vi "Test Assert Not Equal Value.vi"(8 "error in (no error)":errorcluster) -> (0 "error out":errorcluster)   [LabVIEW 2009]
uses:
  classes/Assert/Assert.lvclass
  classes/Test/Test.lvclass
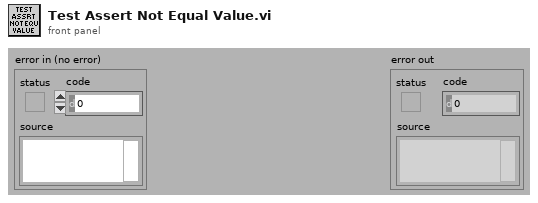
[diagram p1: front panel]
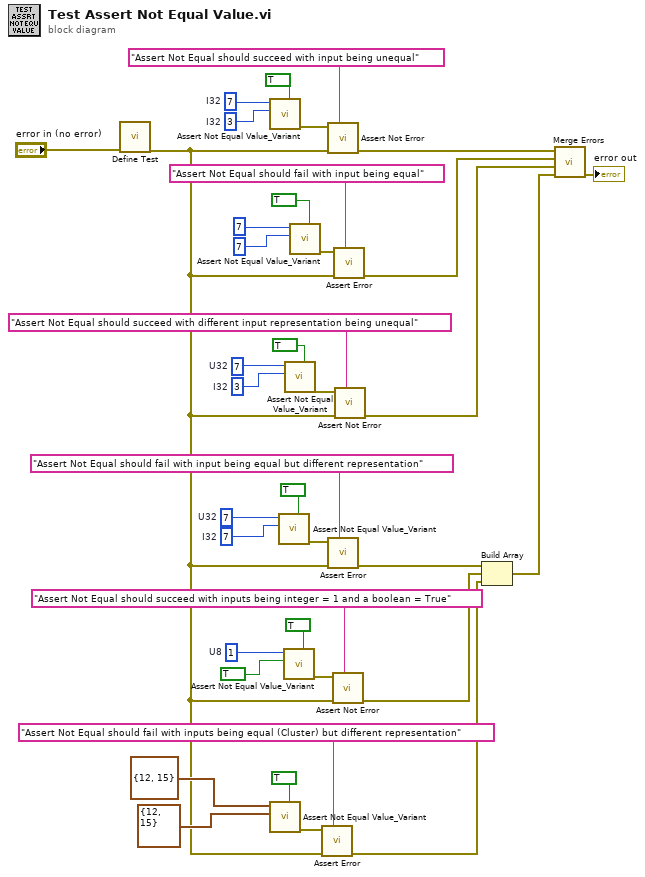
[diagram p0: block diagram]
diagram:
  w12 = u8 1  # U8
  w18 = 7  # I32
  w19 = u32 7  # U32
  w20 = 3  # I32
  w21 = u32 7  # U32
  w28 = 3  # I32
  w29 = 7  # I32
  n1 = call "Define Test.vi"("error in (no error)"="error in (no error)") -> ("error out"=w2:errorcluster)  [unwired: 10 in]
  n2 = call "Assert Not Equal Value_Variant.vi"("Assert Only? (F)"=TRUE, "Y"=w28, "X"=w29) -> ("error out"=w31:errorcluster)  [unwired: 8 in]
  n3 = call "Assert Not Equal Value_Variant.vi"("Assert Only? (F)"=TRUE, "Y"=cluster{"Width":u32, "I32":i32} {"Width"=12, "I32"=15} ("Bounds"), "X"=cluster{"Width":u32, "U32":u32} {"Width"=12, "U32"=15} ("Bounds")) -> ("error out"=w6:errorcluster)  [unwired: 8 in]
  n4 = call "Assert Not Equal Value_Variant.vi"("Assert Only? (F)"=TRUE, "Y"=w18, "X"=w19) -> ("error out"=w15:errorcluster)  [unwired: 8 in]
  n5 = call "Assert Not Equal Value_Variant.vi"("Assert Only? (F)"=TRUE, "Y"=TRUE, "X"=w12) -> ("error out"=w8:errorcluster)  [unwired: 8 in]
  n6 = call "Assert Not Equal Value_Variant.vi"("Assert Only? (F)"=TRUE, "Y"=w20, "X"=w21) -> ("error out"=w23:errorcluster)  [unwired: 8 in]
  n7 = call "Assert Not Equal Value_Variant.vi"("Assert Only? (F)"=TRUE, "Y"=7, "X"=7) -> ("error out"=w27:errorcluster)  [unwired: 8 in]
  n8 = call "Assert Error.vi"("Label"="Assert Not Equal should fail with inputs being equal (Cluster) but different representation", "error in (no error)"=w2, "Error?"=w6) -> ("error out"=w1:errorcluster)  [unwired: 8 in]
  n9 = call "Assert Not Error.vi"("Label"="Assert Not Equal should succeed with input being unequal", "error in (no error)"=w2, "Not Error?"=w31) -> ("error out"=w36:errorcluster)  [unwired: 8 in]
  n10 = call "Assert Error.vi"("Label"="Assert Not Equal should fail with input being equal but different representation", "error in (no error)"=w2, "Error?"=w15) -> ("error out"=w14:errorcluster)  [unwired: 8 in]
  n11 = call "Assert Not Error.vi"("Label"="Assert Not Equal should succeed with inputs being integer = 1 and a boolean = True", "error in (no error)"=w2, "Not Error?"=w8) -> ("error out"=w10:errorcluster)  [unwired: 8 in]
  n12 = call "Assert Error.vi"("Label"="Assert Not Equal should fail with input being equal", "error in (no error)"=w2, "Error?"=w27) -> ("error out"=w37:errorcluster)  [unwired: 8 in]
  n13 = call "Assert Not Error.vi"("Label"="Assert Not Equal should succeed with different input representation being unequal", "error in (no error)"=w2, "Not Error?"=w23) -> ("error out"=w33:errorcluster)  [unwired: 8 in]
  n14 = Build Array(w14, w10, w1) -> (w32:errorcluster[])
  n15 = call <vilib>:"Merge Errors.vi"("error array in"=w32, "error in 3 (no error)"=w33, "error in 2 (no error)"=w37, "error in 1 (no error)"=w36) -> ("error out"=→"error out":errorcluster)  [unwired: 3 in]
